vi "ev3 i2c read.vi"() -> ()   [LabVIEW 2013]
uses:
  <vilib>/NXT/Block Support/HWPage.SensorType.ctl
  <vilib>/NXT/Block Support/HWPage.SensorMode.ctl
  <vilib>/NXT/Block Support/NXT_InputPort.ctl
  <vilib>/NXT/Dual Mode Library/Sensors/i2c_sensors_big.vi
panel:
  out "string":string
  out "Bytes read":u8[](array[numeric])
  in  "Stop Button":bool
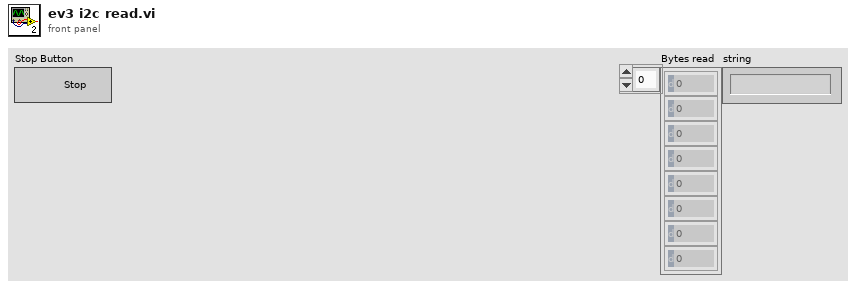
[diagram p1: front panel]
types:
  T1 = typedef "NXT_InputPort.ctl" = u32
  T2 = typedef "HWPage.SensorType.ctl" = u8
  T3 = typedef "HWPage.SensorMode.ctl" = u8
  T4 = typedef "LVHSConnector.ctl" = refnum<class "BrickReference.lvclass">
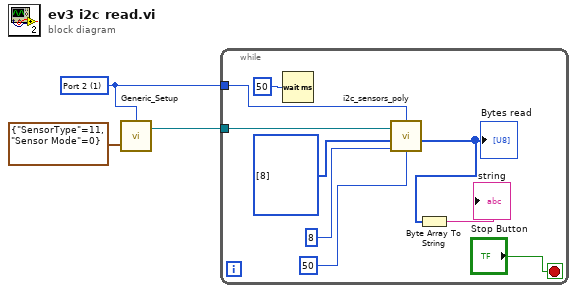
[diagram p0: block diagram]
diagram:
  w1 = T1 1 items=["Port 1", "Port 2", "Port 3", "Port 4"] ("Port")
  n1 = call <vilib>:"Generic_Setup.vi"("Sensor Setup"=cluster{"SensorType":T2, "Sensor Mode":T3} {"SensorType"=11, "Sensor Mode"=0}, "Port"=w1) -> ("NXT/EV3"=w2:T4)  [unwired: 1 in, 1 out]
  n2 = while {
    tunnel: w2 -> [w11]
    tunnel: w1 -> [w10]
    stop <- "Stop Button" stop-if-true
    n3 = Wait (ms)(milliseconds to wait=u32 50) -> ()  [unwired: 1 out]
    n4 = call-poly <vilib>:"i2c_sensors_poly.vi"("Return Length"=u8 8, "Bytes to Write"=u8[] [8], "Wait (msec)"=u32 50, "NXT/EV3"=w11, "Port"=w10) -> ("Bytes read"=w5:u8[])  [unwired: 2 out]
    "Bytes read" <- w5
    n5 = Byte Array To String(unsigned byte array=w5) -> (string=→"string":string)
  }
